vi "testCustomAssertionFailureMessage.vi"() -> ()   [LabVIEW 2019, in "AssertionTest.lvlib" / "AssertNotEquals.lvlib"]
uses:
  AssertNotEquals.lvlib
  Assertion/Assertion.lvlib
  4c0fa4f8-e8bf-466f-afde-48ab27d81456.vi
panel:
  out "error out":errorcluster
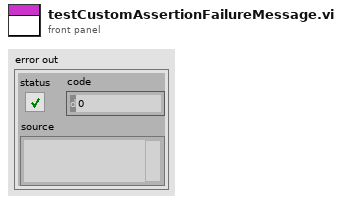
[diagram p1: front panel]
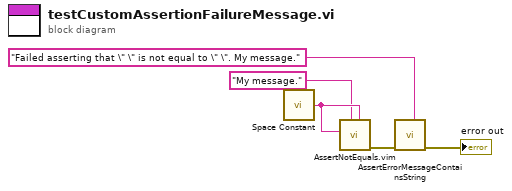
[diagram p0: block diagram]
diagram:
  n1 = call <vilib>:"Space Constant.vi"() -> ("String"=w2:string)
  n2 = call "AssertNotEquals.vim"("Expected"=w2, "Message (\"\")"="My message.", "Actual"=w2) -> ("error out"=w5:errorcluster)  [unwired: 8 in]
  n3 = call "AssertErrorMessageContainsString.vi"("Expected"="Failed asserting that \" \" is not equal to \" \". My message." ("y"), "error in (no error)"=w5) -> ("error out"=→"error out":errorcluster)  [unwired: 9 in]
